vi "CSTK_Icon_Creator_Insert_MainBGColor.vi"(8 "error in (no error)":errorcluster, 9 "主体背景色":u32(colorbox), 11 "图片输入":picture) -> (0 "error out":errorcluster, 3 "图片输出":picture)   [LabVIEW 2015, in "CSTK_Icon Creator.lvlib"]
uses:
  CSTK_Icon Creator.lvlib
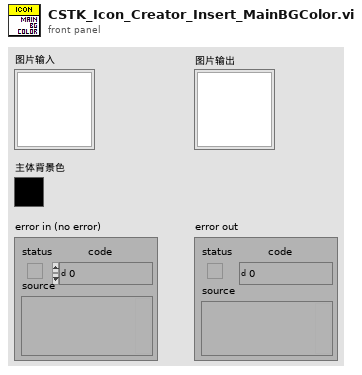
[diagram p1: front panel]
types:
  T1 = typedef "imagedata.ctl" = cluster{"image type":i32, "image depth":i32, "image":u8[], "mask":u8[], "colors":u32[], "Rectangle":cluster{"left":i16, "top":i16, "right":i16, "bottom":i16}}
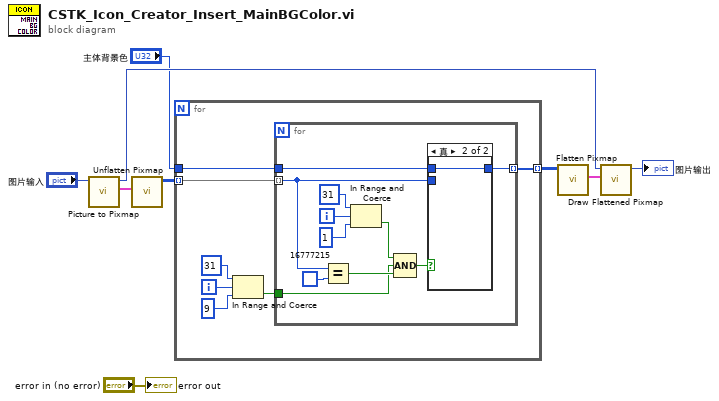
[diagram p0: block diagram]
diagram:
  n1 = call <vilib>:"Picture to Pixmap.vi"("picture"="图片输入") -> ("image data"=w5:T1, "new picture"=w4:picture)  [unwired: 9 in]
  n2 = call <vilib>:"Unflatten Pixmap.vi"("image data"=w5) -> ("24-bit pixmap"=w8:u32[][])  [unwired: 4 in, 6 out]
  n3 = for {
    tunnel: w8 -> [w16] mode=indexing
    tunnel: [w11] -> w6 mode=indexing
    tunnel: "主体背景色" -> [w10]
    i -> [w13]
    n4 = In Range and Coerce(upper limit=31 ("上限"), x=w13, lower limit=9 ("下限")) -> (In Range?=w12:bool)  [unwired: 1 out]
    n5 = for {
      tunnel: w16 -> [w23] mode=indexing
      tunnel: w12 -> [w17]
      tunnel: [w22] -> w11 mode=indexing
      tunnel: w10 -> [w21]
      i -> [w27]
      n6 = Equal?(x=w23, y=u32 16777215) -> (x = y?=w19:bool)
      n7 = In Range and Coerce(upper limit=31 ("上限"), x=w27, lower limit=1 ("下限")) -> (In Range?=w18:bool)  [unwired: 1 out]
      n8 = Compound Arithmetic op=AND ("复合运算")(w18, w17, w19) -> (w20:bool)
      n9 = case shown="真" w20 {
        tunnel: w23 -> [w28 _]
        tunnel: [w28 w29] -> w22
        tunnel: w21 -> [_ w29]
        frame False {
        }
        frame True {
        }
      }
    }
  }
  n10 = call <vilib>:"Flatten Pixmap.vi"("24-bit pixmap"=w6) -> ("image data"=w7:T1)  [unwired: 10 in]
  n11 = call <vilib>:"Draw Flattened Pixmap.vi"("image data"=w7, "picture"=w4) -> ("new picture"=→"图片输出":picture)  [unwired: 7 in]
  "error out" <- "error in (no error)"
